vi "Close.vi"(8 "error in (no error)":errorcluster, 11 "DbConnection in":refnum<class "DbConnection.lvclass">) -> (0 "error out":errorcluster)   [LabVIEW 2020, in "ORM.lvlib" / "DbConnection.lvclass"]
uses:
  DbConnection.lvclass
  DbConnection.lvclass/DbConnection.ctl
  System.Data
  Read connection.vi
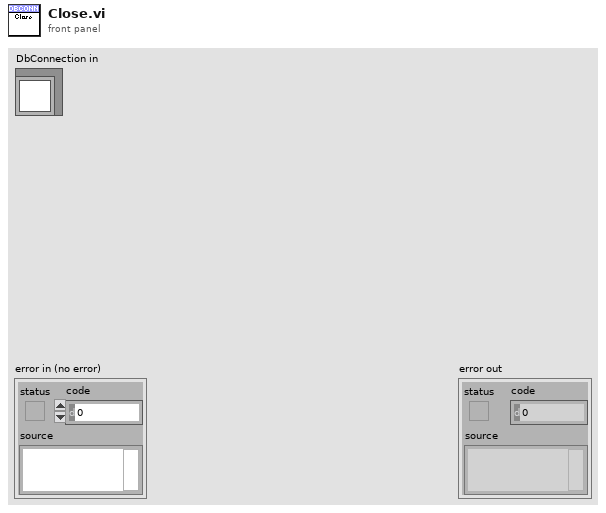
[diagram p1: front panel]
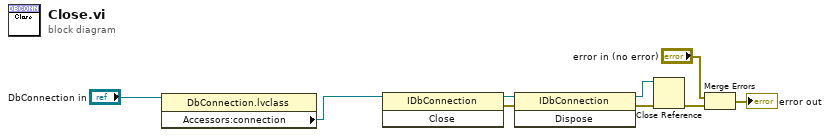
[diagram p0: block diagram]
diagram:
  n1 = property class="DbConnection.lvclass"(reference="DbConnection in") -> ("Accessors:connection"=w1:refnum<k24>)  [unwired: 1 in, 2 out]
  n2 = invoke class="IDbConnection" method="Close"(reference=w1) -> (reference out=w9:refnum<k24>, error out=w6:errorcluster)  [unwired: 2 in, 1 out]
  n3 = invoke class="IDbConnection" method="Dispose"(reference=w9, error in=w6) -> (reference out=w7:refnum<k24>, error out=w8:errorcluster)  [unwired: 1 in, 1 out]
  n4 = Close Reference(reference=w7, error in (no error)=w8) -> (error out=w5:errorcluster)
  n5 = Merge Errors("error in (no error)", w5) -> (→"error out":errorcluster)
